vi "SMU 2450 main.vi"(8 "update time (100ms)":u32=100, 10 "Mailbox address Top":T2, 11 "Module mailbox":T2) -> (1 "SMU status":T1 {"Measure Function" items=["Volts", "Current", "Auto Resistance", "Manual Resistance", "Digitize Voltage", "Digitize Current"]; "Source Mode" items=["Voltage", "Current"]}, 3 "Ended":bool)   [LabVIEW 2021, in "Source meter.lvlib"]
doc: "Module for general use of SMU 2450."
uses:
  Source meter.lvlib
  Messenger service/Data types/Mailbox address.ctl
  ctls/SMU status.ctl
  Messenger service/Data types/Module name.ctl
  ctls/SMU settings.ctl
  ctls/MSG to SMU.ctl
  ctls/SMU Commands.ctl
  <userlib>/_MGI/1D Array/MGI Average/MGI Average (DBL[]).vi
  <instrlib>/Keithley 2450/Keithley 2450.lvlib
  Messenger service/MessengerLib.lvlib
panel:
  out "error IO":errorcluster
  out "Unread":i32
  out "time ms":u32
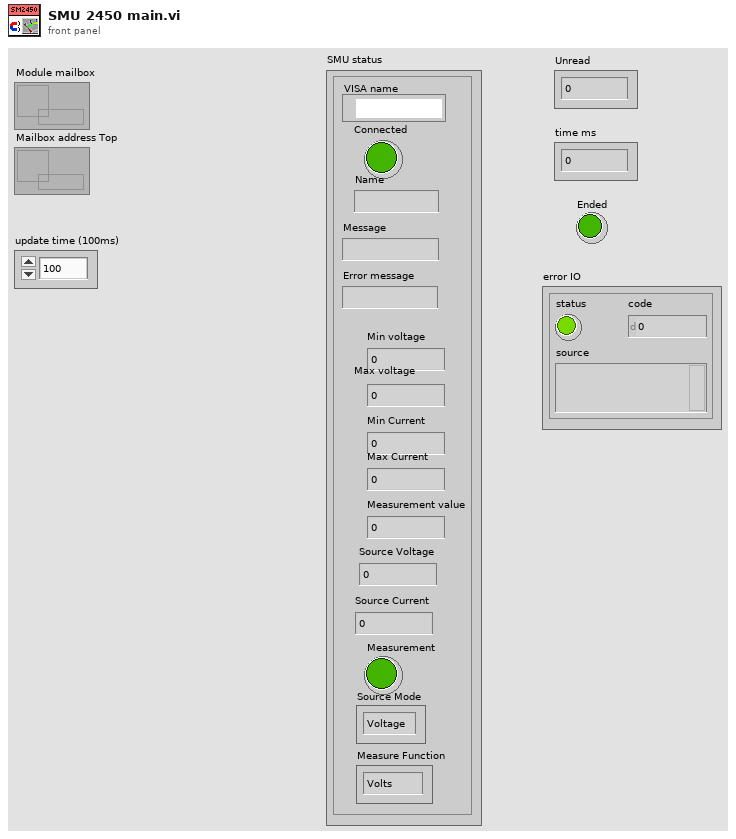
[diagram p1: front panel]
types:
  T1 = typedef "Source meter.lvlib/SMU status.ctl" = cluster{"VISA name":refnum<visa-resource-name>, "Connected":bool, "Name":string, "Message":string, "Error message":string, "Min voltage":dbl, "Max voltage":dbl, "Min Current":dbl, "Max Current":dbl, "Measurement value":dbl, "Source Voltage":dbl, "Measurement":bool, "Source Current":dbl, "Source Mode":u16, "Measure Function":u16}
  T2 = typedef "MessengerLib.lvlib/Mailbox address.ctl" = refnum<queue>
  T3 = typedef "Source meter.lvlib/MSG to SMU.ctl" = cluster{"Command":T4, "Data":variant}
  T4 = typedef "Source meter.lvlib/SMU Commands.ctl" = enum16{"Ignore", "Connect", "Update", "Set measurement", "Start measurement", "Get actual results", "Stop measurement", "Disconnect", "End"}
  T5 = typedef "MessengerLib.lvlib/Module name.ctl" = enum16{"Emty", "Magnet", "VTI", "Excitation", "Servo", "Acquisition", "Rotator", "Digitizer", "SMU2450", "Carousel", "Multimeter", "Tmp monitor", "Power monitor"}
  T6 = typedef "Source meter.lvlib/SMU settings.ctl" = cluster{"Source Mode ":u16, "Source Level":dbl, "Source Limit":dbl, "Measure Function":u16, "Remote sense":bool, "Clear buffer?":bool, "Beep":bool, "High Capacity":bool, "Terminals":u16, "PLCs":dbl, "Fast measurement":bool}
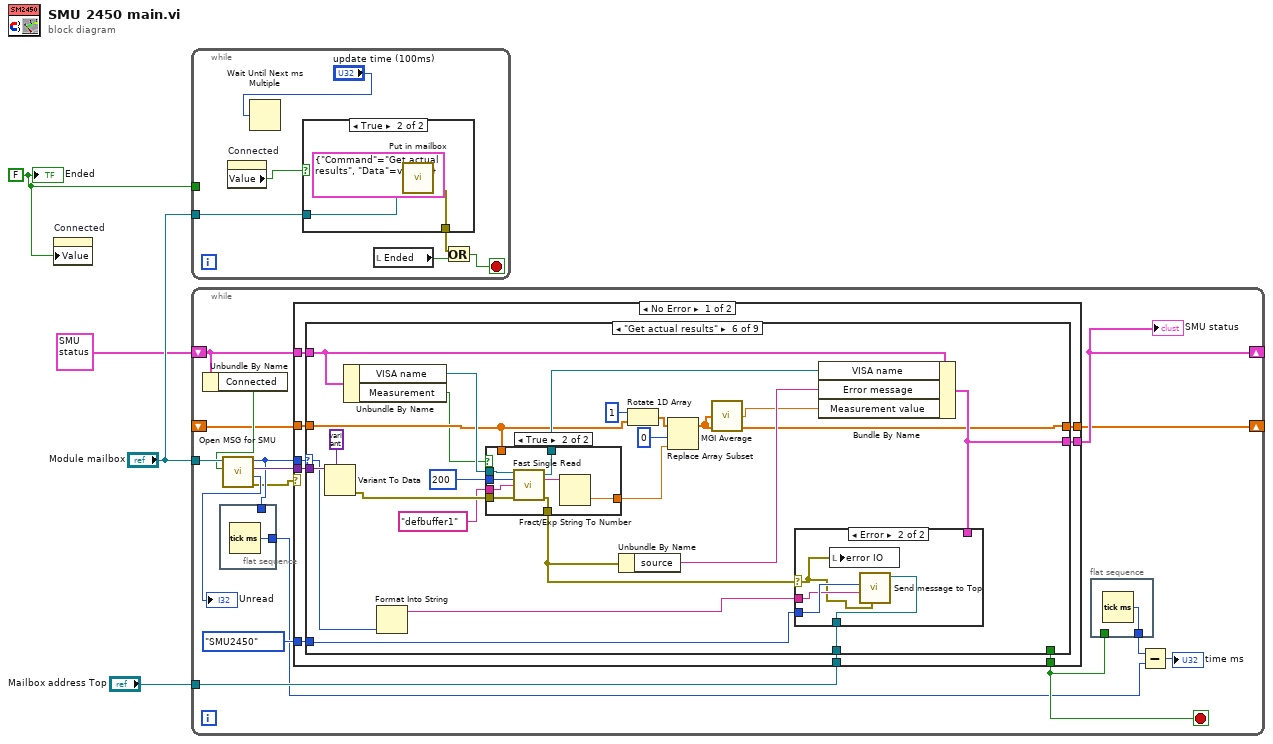
[diagram p0: block diagram]
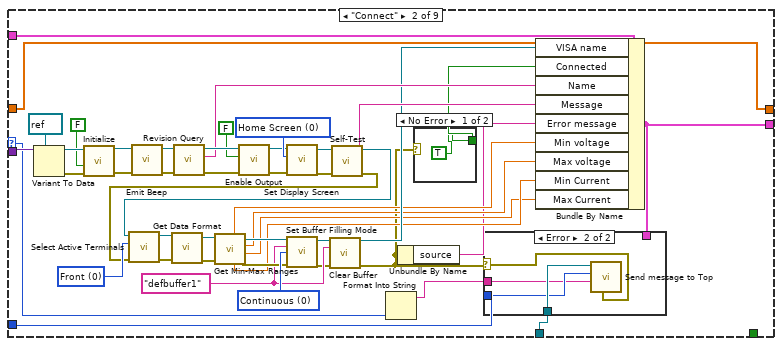
[diagram p4: hidden frame]
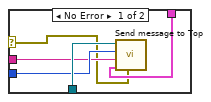
[diagram p6: hidden frame]
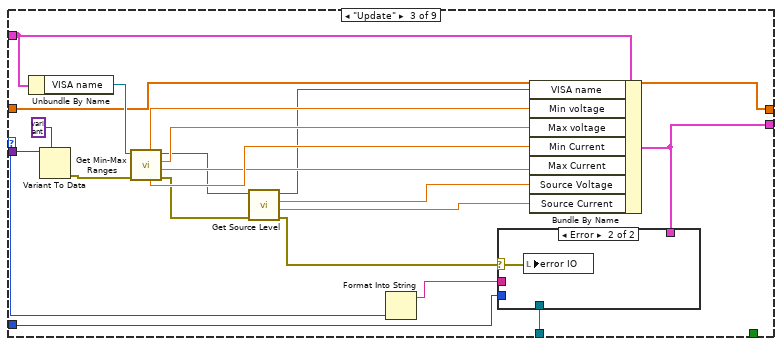
[diagram p7: hidden frame]
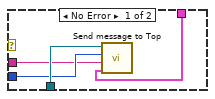
[diagram p8: hidden frame]
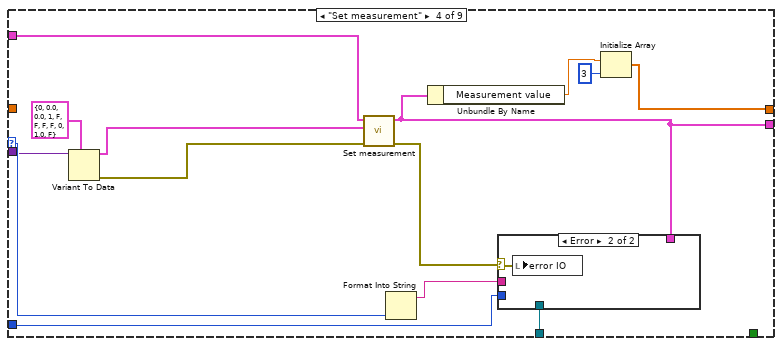
[diagram p9: hidden frame]
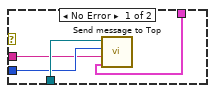
[diagram p10: hidden frame]
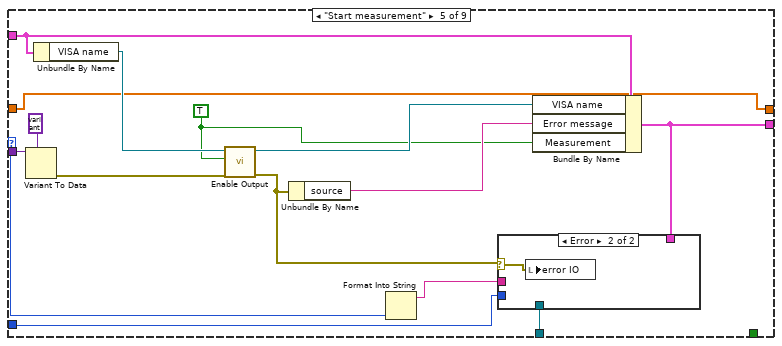
[diagram p11: hidden frame]
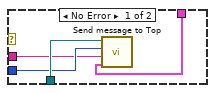
[diagram p12: hidden frame]
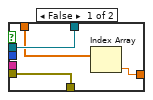
[diagram p13: hidden frame]
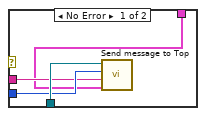
[diagram p14: hidden frame]
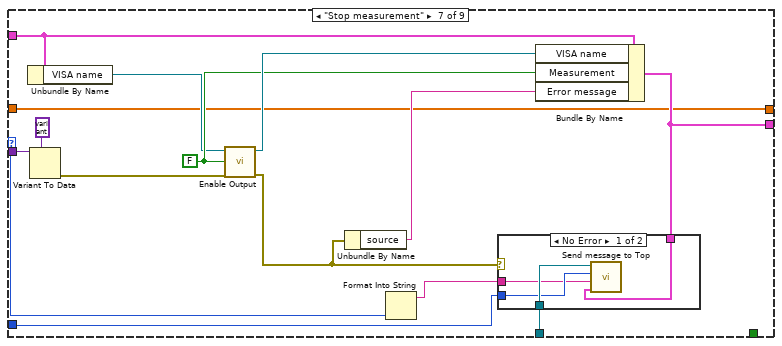
[diagram p15: hidden frame]
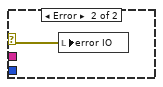
[diagram p16: hidden frame]
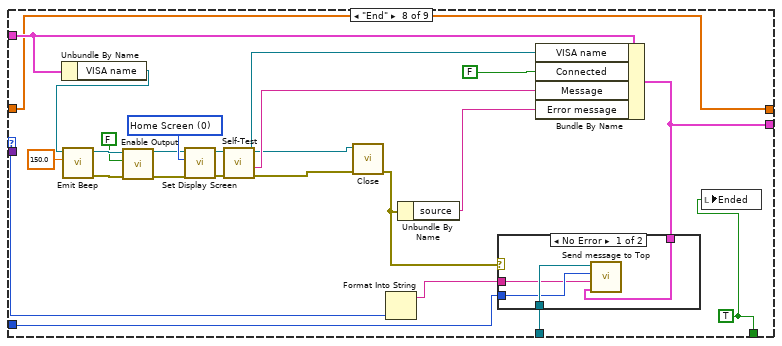
[diagram p17: hidden frame]
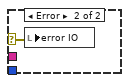
[diagram p18: hidden frame]
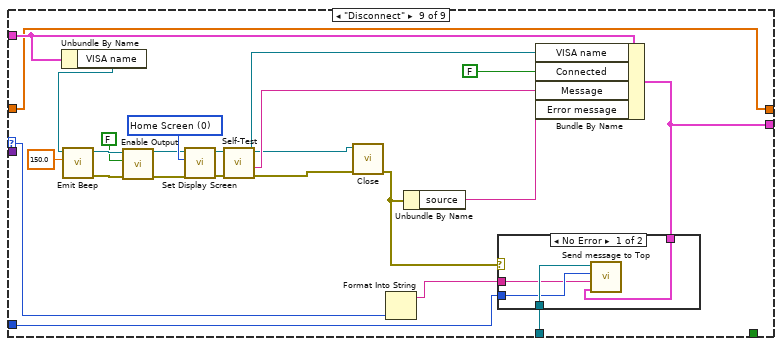
[diagram p19: hidden frame]
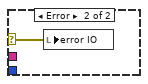
[diagram p20: hidden frame]
diagram:
  w1 = FALSE ("Ended")
  n1 = property on="Connected" class="Bool (strict)"("Value"=w1) -> ()  [unwired: 2 in, 2 out]
  n2 = while {
    tunnel: w1 -> [_]
    tunnel: "Module mailbox" -> [w6]
    stop <- w8 stop-if-true
    n3 = property on="Connected" class="Bool (strict)"() -> ("Value"=w5:bool)  [unwired: 2 in, 2 out]
    n4 = Wait Until Next ms Multiple(millisecond multiple="update time (100ms)") -> ()  [unwired: 1 out]
    n5 = case shown="True" w5 {
      tunnel: [_ w12] -> w7
      tunnel: w6 -> [_ w11]
      frame False {
      }
      frame True {
        n6 = call "Put in mailbox.vi"("Message"=T3 {"Command"=enum."Get actual results", "Data"=variant} ("MSG to Source meter"), "Queue in"=w11) -> ("error out"=w12:errorcluster)  [unwired: 7 in, 2 out]
      }
    }
    n7 = local read "Ended"() -> (w9:bool)
    n8 = Or(x=w7, y=w9) -> (x .or. y?=w8:bool)
  }
  n9 = while {
    tunnel: "Module mailbox" -> [w29]
    tunnel: "Mailbox address Top" -> [w27]
    shift-right: [w25] -> _
    shift-left: T1 {"VISA name"="", "Connected"=FALSE, "Name"="", "Message"="", "Error message"="", "Min voltage"=0.0, "Max voltage"=0.0, "Min Current"=0.0, "Max Current"=0.0, "Measurement value"=0.0, "Source Voltage"=0.0, "Measurement"=FALSE, "Source Current"=0.0, "Source Mode"=0, "Measure Function"=0} ("SMU status") -> [w24]
    shift-right: [w15] -> _
    shift-left: _ -> [w14]
    stop <- w21 stop-if-true
    n10 = Unbundle By Name(w24) -> ("Connected"=w23:bool)
    n11 = flat-sequence {
      tunnel: w22 -> [_]
      tunnel: [w287] -> w19
      frame #0 {
        n12 = Tick Count (ms)() -> (millisecond timer value=w287:u32)
      }
    }
    n13 = call "Open MSG for SMU.vi"("Initialized"=w23, "Queue in"=w29) -> ("error out"=w16:errorcluster, "Unread"=→"Unread":i32, "Data"=w28:variant, "Command"=w22:T4)  [unwired: 6 in]
    n14 = case shown="No Error" w16 {
      selector: w16 -> [_ w286]
      tunnel: w28 -> [w38 _]
      tunnel: w27 -> [w37 _]
      tunnel: Module_name."SMU2450" ("Module") -> [w36 _]
      tunnel: [w35 w285] -> w25
      tunnel: w24 -> [w34 w285]
      tunnel: w22 -> [w33 _]
      tunnel: [w32 FALSE] -> w21
      tunnel: [w31 w283] -> w15
      tunnel: w14 -> [w30 w283]
      frame No Error {
        n15 = case shown="\"Get actual results\"" w33 {
          selector: w33 -> [_ w53 w115 w134 w154 w182 w217 w236 w265]
          tunnel: w38 -> [_ w87 w118 w130 w157 w185 w220 _ _]
          tunnel: w34 -> [w40 w75 w112 w132 w150 w175 w214 w232 w262]
          tunnel: w37 -> [_ w55 w117 w136 w156 w184 w219 w238 w267]
          tunnel: w36 -> [_ w54 w116 w135 w155 w183 w218 w237 w266]
          tunnel: [w40 w48 w114 w127 w153 w181 w216 w235 w264] -> w35
          tunnel: [_ _ _ _ _ _ _ w227 _] -> w32
          tunnel: [w39 w41 w98 w124 w143 w167 w206 w226 w255] -> w31
          tunnel: w30 -> [w39 w41 w98 _ w143 w164 w206 w226 w255]
          frame "Ignore", Default {
          }
          frame "Connect" {
            w58 = "defbuffer1" ("Buffer Name (defbuffer1)")
            w80 = u16 0 items=["Front", "Rear"] ("Active Terminals (0: Front)")
            w81 = u16 0 items=["Home Screen", "Source Screen", "Plot Screen", "User-defined Screen", "Statistics Screen", "Settings Screen", "Graph Screen", "Data sheet Screen"] ("Screen Home")
            w83 = u16 0 items=["Continuous", "Once"] ("Fill Type")
            n16 = Variant To Data(type=refnum<visa-resource-name> refnum ("VISA resource name"), Variant=w87) -> (data=w85:refnum<visa-resource-name>, error out=w84:errorcluster)  [unwired: 1 in]
            n17 = call <instrlib>:"Initialize.vi"("error in (no error)"=w84, "Reset (True)"=FALSE, "VISA resource name"=w85) -> ("error out"=w78:errorcluster, "VISA resource name out"=w79:refnum<visa-resource-name>)  [unwired: 7 in]
            n18 = call <instrlib>:"Emit Beep.vi"("error in (no error)"=w78, "VISA resource name"=w79) -> ("error out"=w76:errorcluster, "VISA resource name out"=w77:refnum<visa-resource-name>)  [unwired: 8 in]
            n19 = call <instrlib>:"Revision Query.vi"("error in (no error)"=w76, "VISA resource name"=w77) -> ("error out"=w73:errorcluster, "Instrument Driver Revision"=w72:string, "VISA resource name out"=w74:refnum<visa-resource-name>)  [unwired: 6 in, 1 out]
            n20 = call <instrlib>:"Enable Output.vi"("error in (no error)"=w73, "Enable Output (T: Enable)"=FALSE, "VISA resource name"=w74) -> ("error out"=w69:errorcluster, "VISA resource name out"=w70:refnum<visa-resource-name>)  [unwired: 7 in]
            n21 = call <instrlib>:"Set Display Screen.vi"("error in (no error)"=w69, "Screen Home"=w81, "VISA resource name"=w70) -> ("error out"=w66:errorcluster, "VISA resource name out"=w67:refnum<visa-resource-name>)  [unwired: 7 in]
            n22 = call <instrlib>:"Self-Test.vi"("error in (no error)"=w66, "VISA resource name"=w67) -> ("error out"=w44:errorcluster, "Self-Test Result Message"=w68:string, "VISA resource name out"=w45:refnum<visa-resource-name>)  [unwired: 6 in, 1 out]
            n23 = call <instrlib>:"Select Active Terminals.vi"("error in (no error)"=w44, "Active Terminals (0: Front)"=w80, "VISA resource name"=w45) -> ("error out"=w64:errorcluster, "VISA resource name out"=w65:refnum<visa-resource-name>)  [unwired: 7 in]
            n24 = call <instrlib>:"Get Data Format.vi"("VISA resource name"=w65, "error in (no error)"=w64) -> ("VISA resource name out"=w63:refnum<visa-resource-name>, "error out"=w62:errorcluster)  [unwired: 11 in, 1 out]
            n25 = call <instrlib>:"Get Min-Max Ranges.vi"("error in (no error)"=w62, "VISA resource name"=w63) -> ("error out"=w60:errorcluster, "I Max"=w49:dbl, "V Max"=w51:dbl, "VISA resource name out"=w61:refnum<visa-resource-name>, "I Min"=w50:dbl, "V Min"=w52:dbl)  [unwired: 4 in]
            n26 = call <instrlib>:"Set Buffer Filling Mode.vi"("VISA resource name"=w61, "Buffer Name (defbuffer1)"=w58, "Fill Type"=w83, "error in (no error)"=w60) -> ("VISA resource name out"=w59:refnum<visa-resource-name>, "error out"=w57:errorcluster)  [unwired: 10 in]
            n27 = call <instrlib>:"Clear Buffer.vi"("VISA resource name"=w59, "Buffer Name (defbuffer1)"=w58, "error in (no error)"=w57) -> ("VISA resource name out"=w56:refnum<visa-resource-name>, "error out"=w43:errorcluster)  [unwired: 11 in]
            n28 = Format Into String(w53) -> (resulting string=w47:string)  [unwired: 3 in, 1 out]
            n29 = Unbundle By Name(w43) -> ("source"=w46:string)
            n30 = case shown="No Error" w43 {
              tunnel: [TRUE ("Connected") _] -> w42
              frame No Error {
              }
              frame Error {
              }
            }
            n31 = Bundle By Name(cluster=w75, "VISA name"=w56, "Connected"=w42, "Name"=w72, "Message"=w68, "Error message"=w46, "Min voltage"=w52, "Max voltage"=w51, "Min Current"=w50, "Max Current"=w49) -> (w48:T1)
            n32 = case shown="Error" w43 {
              selector: w43 -> [w89 w94]
              tunnel: w55 -> [w93 w97]
              tunnel: w54 -> [w92 w96]
              tunnel: w48 -> [w91 _]
              tunnel: w47 -> [w90 w95]
              frame No Error {
                n33 = call "Send message to Top.vi"("Error in (no error)"=w89, "Data"=w91, "Response"=w90, "Module"=w92, "Mailbox address in"=w93) -> ()  [unwired: 5 in, 2 out]
              }
              frame Error {
                n34 = call "Send message to Top.vi"("Error in (no error)"=w94, "Response"=w95, "Module"=w96, "Mailbox address in"=w97) -> ()  [unwired: 6 in, 2 out]
              }
            }
          }
          frame "Update" {
            n35 = Unbundle By Name(w112) -> ("VISA name"=w110:refnum<visa-resource-name>)
            n36 = Variant To Data(type=variant, Variant=w118) -> (error out=w111:errorcluster)  [unwired: 1 in, 1 out]
            n37 = call <instrlib>:"Get Min-Max Ranges.vi"("error in (no error)"=w111, "VISA resource name"=w110) -> ("error out"=w102:errorcluster, "I Max"=w105:dbl, "V Max"=w107:dbl, "VISA resource name out"=w104:refnum<visa-resource-name>, "I Min"=w106:dbl, "V Min"=w108:dbl)  [unwired: 4 in]
            n38 = call <instrlib>:"Get Source Level.vi"("error in (no error)"=w102, "VISA resource name"=w104) -> ("error out"=w101:errorcluster, "Current Level Out"=w100:dbl, "Voltage Level Out"=w99:dbl, "VISA resource name out"=w103:refnum<visa-resource-name>)  [unwired: 6 in]
            n39 = Format Into String(w115) -> (resulting string=w113:string)  [unwired: 3 in, 1 out]
            n40 = Bundle By Name(cluster=w112, "VISA name"=w103, "Min voltage"=w108, "Max voltage"=w107, "Min Current"=w106, "Max Current"=w105, "Source Voltage"=w99, "Source Current"=w100) -> (w114:T1)
            n41 = case shown="Error" w101 {
              selector: w101 -> [_ w123]
              tunnel: w117 -> [w122 _]
              tunnel: w116 -> [w121 _]
              tunnel: w114 -> [w120 _]
              tunnel: w113 -> [w119 _]
              frame No Error {
                n42 = call "Send message to Top.vi"("Data"=w120, "Response"=w119, "Module"=w121, "Mailbox address in"=w122) -> ()  [unwired: 6 in, 2 out]
              }
              frame Error {
                n43 = local write "error IO"(w123) -> ()
              }
            }
          }
          frame "Set measurement" {
            n44 = Variant To Data(type=T6 {"Source Mode "=0, "Source Level"=0.0, "Source Limit"=0.0, "Measure Function"=1, "Remote sense"=FALSE, "Clear buffer?"=FALSE, "Beep"=FALSE, "High Capacity"=FALSE, "Terminals"=0, "PLCs"=1.0, "Fast measurement"=FALSE}, Variant=w130) -> (data=w129:T6, error out=w128:errorcluster)  [unwired: 1 in]
            n45 = call "Set measurement.vi"("error in (no error)"=w128, "Measurement settings"=w129, "SMU status in"=w132) -> ("error out"=w137:errorcluster, "SMU status out"=w127:T1)  [unwired: 7 in]
            n46 = Format Into String(w134) -> (resulting string=w133:string)  [unwired: 3 in, 1 out]
            n47 = Unbundle By Name(w127) -> ("Measurement value"=w125:dbl)
            n48 = case shown="Error" w137 {
              selector: w137 -> [_ w142]
              tunnel: w136 -> [w141 _]
              tunnel: w135 -> [w140 _]
              tunnel: w127 -> [w139 _]
              tunnel: w133 -> [w138 _]
              frame No Error {
                n49 = call "Send message to Top.vi"("Data"=w139, "Response"=w138, "Module"=w140, "Mailbox address in"=w141) -> ()  [unwired: 6 in, 2 out]
              }
              frame Error {
                n50 = local write "error IO"(w142) -> ()
              }
            }
            n51 = Initialize Array(w125, 3 ("dimension size")) -> (w124:dbl[])
          }
          frame "Start measurement" {
            w144 = TRUE ("Enable Output (T: Enable)")
            n52 = Variant To Data(type=variant, Variant=w157) -> (error out=w148:errorcluster)  [unwired: 1 in, 1 out]
            n53 = Unbundle By Name(w150) -> ("VISA name"=w147:refnum<visa-resource-name>)
            n54 = call <instrlib>:"Enable Output.vi"("error in (no error)"=w148, "Enable Output (T: Enable)"=w144, "VISA resource name"=w147) -> ("error out"=w149:errorcluster, "VISA resource name out"=w145:refnum<visa-resource-name>)  [unwired: 7 in]
            n55 = Unbundle By Name(w149) -> ("source"=w151:string)
            n56 = Format Into String(w154) -> (resulting string=w152:string)  [unwired: 3 in, 1 out]
            n57 = Bundle By Name(cluster=w150, "VISA name"=w145, "Error message"=w151, "Measurement"=w144) -> (w153:T1)
            n58 = case shown="Error" w149 {
              selector: w149 -> [_ w162]
              tunnel: w156 -> [w161 _]
              tunnel: w155 -> [w160 _]
              tunnel: w153 -> [w159 _]
              tunnel: w152 -> [w158 _]
              frame No Error {
                n59 = call "Send message to Top.vi"("Data"=w159, "Response"=w158, "Module"=w160, "Mailbox address in"=w161) -> ()  [unwired: 6 in, 2 out]
              }
              frame Error {
                n60 = local write "error IO"(w162) -> ()
              }
            }
          }
          frame "Get actual results" {
            n61 = Variant To Data(type=variant, Variant=w185) -> (error out=w179:errorcluster)  [unwired: 1 in, 1 out]
            n62 = Unbundle By Name(w175) -> ("VISA name"=w174:refnum<visa-resource-name>, "Measurement"=w163:bool)
            n63 = Format Into String(w182) -> (resulting string=w180:string)  [unwired: 3 in, 1 out]
            n64 = case shown="True" w163 {
              tunnel: w179 -> [w189 w197]
              tunnel: [w188 w196] -> w178
              tunnel: 200 ("Timeout (10000 ms)") -> [_ w195]
              tunnel: "defbuffer1" ("Buffer Name (defbuffer1)") -> [_ w194]
              tunnel: w174 -> [w188 w192]
              tunnel: [w189 w191] -> w173
              tunnel: [w187 w190] -> w166
              tunnel: w164 -> [w186 _]
              frame False {
                n65 = Index Array(array=w186) -> (element=w187:dbl)  [unwired: 1 in]
              }
              frame True {
                n66 = call "Fast Single Read.vi"("VISA resource name"=w192, "Timeout (10000 ms)"=w195, "Buffer Name (defbuffer1)"=w194, "error in (no error)"=w197) -> ("VISA resource name out"=w196:refnum<visa-resource-name>, "Data out"=w193:string, "error out"=w191:errorcluster)  [unwired: 9 in]
                n67 = Fract/Exp String To Number(string=w193) -> (number=w190:dbl)  [unwired: 3 in, 1 out]
              }
            }
            n68 = Unbundle By Name(w173) -> ("source"=w172:string)
            n69 = Rotate 1D Array(1:w164, 2:1 ("n")) -> (0:w168:dbl[])
            n70 = Replace Array Subset(array=w168, new element=w166, index=0) -> (w167:dbl[])
            n71 = call-poly <userlib>:"MGI Average.vi"("Double[]"=w167) -> ("Average"=w169:dbl)  [unwired: 1 in]
            n72 = Bundle By Name(cluster=w175, "VISA name"=w178, "Error message"=w172, "Measurement value"=w169) -> (w181:T1)
            n73 = case shown="Error" w173 {
              selector: w173 -> [_ w202]
              tunnel: w184 -> [w201 w205]
              tunnel: w183 -> [w200 w204]
              tunnel: w181 -> [w198 _]
              tunnel: w180 -> [w199 w203]
              frame No Error {
                n74 = call "Send message to Top.vi"("Data"=w198, "Response"=w199, "Module"=w200, "Mailbox address in"=w201) -> ()  [unwired: 6 in, 2 out]
              }
              frame Error {
                n75 = local write "error IO"(w202) -> ()
                n76 = call "Send message to Top.vi"("Error in (no error)"=w202, "Response"=w203, "Module"=w204, "Mailbox address in"=w205) -> ()  [unwired: 6 in, 2 out]
              }
            }
          }
          frame "Stop measurement" {
            w211 = FALSE ("Enable Output (T: Enable)")
            n77 = Unbundle By Name(w214) -> ("VISA name"=w208:refnum<visa-resource-name>)
            n78 = Variant To Data(type=variant, Variant=w220) -> (error out=w213:errorcluster)  [unwired: 1 in, 1 out]
            n79 = call <instrlib>:"Enable Output.vi"("error in (no error)"=w213, "Enable Output (T: Enable)"=w211, "VISA resource name"=w208) -> ("error out"=w210:errorcluster, "VISA resource name out"=w212:refnum<visa-resource-name>)  [unwired: 7 in]
            n80 = Unbundle By Name(w210) -> ("source"=w209:string)
            n81 = Format Into String(w217) -> (resulting string=w215:string)  [unwired: 3 in, 1 out]
            n82 = Bundle By Name(cluster=w214, "VISA name"=w212, "Measurement"=w211, "Error message"=w209) -> (w216:T1)
            n83 = case shown="No Error" w210 {
              selector: w210 -> [_ w225]
              tunnel: w219 -> [w224 _]
              tunnel: w218 -> [w223 _]
              tunnel: w216 -> [w222 _]
              tunnel: w215 -> [w221 _]
              frame No Error {
                n84 = call "Send message to Top.vi"("Data"=w222, "Response"=w221, "Module"=w223, "Mailbox address in"=w224) -> ()  [unwired: 6 in, 2 out]
              }
              frame Error {
                n85 = local write "error IO"(w225) -> ()
              }
            }
          }
          frame "End" {
            w227 = TRUE
            w249 = u16 0 items=["Home Screen", "Source Screen", "Plot Screen", "User-defined Screen", "Statistics Screen", "Settings Screen", "Graph Screen", "Data sheet Screen"] ("Screen Home")
            n86 = Unbundle By Name(w232) -> ("VISA name"=w231:refnum<visa-resource-name>)
            n87 = call <instrlib>:"Emit Beep.vi"("Beep Frequency (300)"=150.0, "VISA resource name"=w231) -> ("error out"=w247:errorcluster, "VISA resource name out"=w248:refnum<visa-resource-name>)  [unwired: 8 in]
            n88 = call <instrlib>:"Enable Output.vi"("error in (no error)"=w247, "Enable Output (T: Enable)"=FALSE, "VISA resource name"=w248) -> ("error out"=w243:errorcluster, "VISA resource name out"=w244:refnum<visa-resource-name>)  [unwired: 7 in]
            n89 = call <instrlib>:"Set Display Screen.vi"("error in (no error)"=w243, "Screen Home"=w249, "VISA resource name"=w244) -> ("error out"=w240:errorcluster, "VISA resource name out"=w241:refnum<visa-resource-name>)  [unwired: 7 in]
            n90 = call <instrlib>:"Self-Test.vi"("error in (no error)"=w240, "VISA resource name"=w241) -> ("error out"=w233:errorcluster, "Self-Test Result Message"=w242:string, "VISA resource name out"=w239:refnum<visa-resource-name>)  [unwired: 6 in, 1 out]
            n91 = call <instrlib>:"Close.vi"("error in (no error)"=w233, "VISA resource name"=w239) -> ("error out"=w230:errorcluster)  [unwired: 9 in]
            n92 = Format Into String(w236) -> (resulting string=w234:string)  [unwired: 3 in, 1 out]
            n93 = Unbundle By Name(w230) -> ("source"=w229:string)
            n94 = Bundle By Name(cluster=w232, "VISA name"=w239, "Connected"=FALSE, "Message"=w242, "Error message"=w229) -> (w235:T1)
            n95 = case shown="No Error" w230 {
              selector: w230 -> [_ w254]
              tunnel: w238 -> [w253 _]
              tunnel: w237 -> [w252 _]
              tunnel: w235 -> [w251 _]
              tunnel: w234 -> [w250 _]
              frame No Error {
                n96 = call "Send message to Top.vi"("Data"=w251, "Response"=w250, "Module"=w252, "Mailbox address in"=w253) -> ()  [unwired: 6 in, 2 out]
              }
              frame Error {
                n97 = local write "error IO"(w254) -> ()
              }
            }
            n98 = local write "Ended"(w227) -> ()
          }
          frame "Disconnect" {
            w277 = u16 0 items=["Home Screen", "Source Screen", "Plot Screen", "User-defined Screen", "Statistics Screen", "Settings Screen", "Graph Screen", "Data sheet Screen"] ("Screen Home")
            n99 = Unbundle By Name(w262) -> ("VISA name"=w261:refnum<visa-resource-name>)
            n100 = call <instrlib>:"Emit Beep.vi"("Beep Frequency (300)"=150.0, "VISA resource name"=w261) -> ("error out"=w275:errorcluster, "VISA resource name out"=w276:refnum<visa-resource-name>)  [unwired: 8 in]
            n101 = call <instrlib>:"Enable Output.vi"("error in (no error)"=w275, "Enable Output (T: Enable)"=FALSE, "VISA resource name"=w276) -> ("error out"=w271:errorcluster, "VISA resource name out"=w272:refnum<visa-resource-name>)  [unwired: 7 in]
            n102 = call <instrlib>:"Set Display Screen.vi"("error in (no error)"=w271, "Screen Home"=w277, "VISA resource name"=w272) -> ("error out"=w268:errorcluster, "VISA resource name out"=w269:refnum<visa-resource-name>)  [unwired: 7 in]
            n103 = call <instrlib>:"Self-Test.vi"("error in (no error)"=w268, "VISA resource name"=w269) -> ("error out"=w260:errorcluster, "Self-Test Result Message"=w270:string, "VISA resource name out"=w259:refnum<visa-resource-name>)  [unwired: 6 in, 1 out]
            n104 = call <instrlib>:"Close.vi"("error in (no error)"=w260, "VISA resource name"=w259) -> ("error out"=w258:errorcluster)  [unwired: 9 in]
            n105 = Format Into String(w265) -> (resulting string=w263:string)  [unwired: 3 in, 1 out]
            n106 = Unbundle By Name(w258) -> ("source"=w257:string)
            n107 = Bundle By Name(cluster=w262, "VISA name"=w259, "Connected"=FALSE, "Message"=w270, "Error message"=w257) -> (w264:T1)
            n108 = case shown="No Error" w258 {
              selector: w258 -> [_ w282]
              tunnel: w267 -> [w281 _]
              tunnel: w266 -> [w280 _]
              tunnel: w264 -> [w279 _]
              tunnel: w263 -> [w278 _]
              frame No Error {
                n109 = call "Send message to Top.vi"("Data"=w279, "Response"=w278, "Module"=w280, "Mailbox address in"=w281) -> ()  [unwired: 6 in, 2 out]
              }
              frame Error {
                n110 = local write "error IO"(w282) -> ()
              }
            }
          }
        }
      }
      frame Error {
        "error IO" <- w286
      }
    }
    "SMU status" <- w25
    n111 = flat-sequence {
      tunnel: w21 -> [_]
      tunnel: [w288] -> w20
      frame #0 {
        n112 = Tick Count (ms)() -> (millisecond timer value=w288:u32)
      }
    }
    n113 = Subtract(x=w20, y=w19) -> (x-y=→"time ms":u32)
  }
  "Ended" <- w1
